vi "GT Get Crd Buffer Mode.vi"(7 "fifo":i16, 8 "error in (no error)":errorcluster caption="错误输入（无错误）", 9 "pStaticMode":i16, 10 "crd":i16, 11 "cardNum":i16) -> (0 "error out":errorcluster caption="错误输出", 1 "pStaticMode out":i16, 3 "function return":i16)   [LabVIEW 2020, in "gts.lvlib"]
doc: "GT_API GT_GetCrdBufferMode(short cardNum,short crd,short *pStaticMode,short fifo);"
uses:
  gts.lvlib
  dll/32bit/multi_card/gts.dll
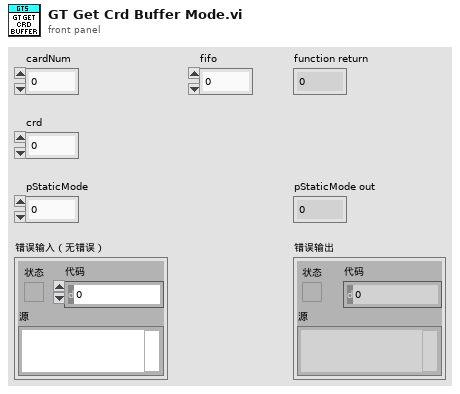
[diagram p1: front panel]
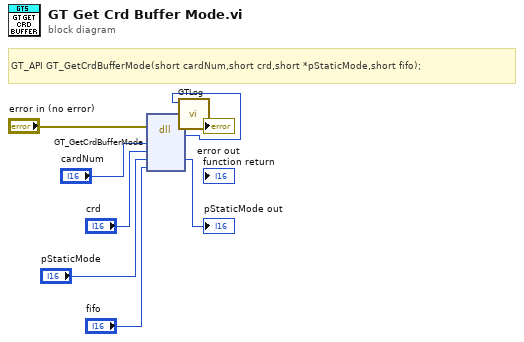
[diagram p0: block diagram]
diagram:
  # "GT_API GT_GetCrdBufferMode(short cardNum,short crd,short *pStaticMode,short fifo);"
  n1 = dll-call lib="C:/1228/dll/32bit/multi_card/gts.dll" fn="GT_GetCrdBufferMode"(error in="error in (no error)", "cardNum"="cardNum", "crd"="crd", "pStaticMode"="pStaticMode", "fifo"="fifo") -> (error out=w3:errorcluster, w1:i16, "pStaticMode"=→"pStaticMode out":i16)  [unwired: 5 in, 1 out]
  n2 = call "GTLog.vi"("error in (no error)"=w3, "Numeric"=w1) -> ("error out"=→"error out":errorcluster)  [unwired: 9 in]
